vi "Set RfsaWlan Handle.vi"(8 "error in (no error)":errorcluster, 10 "RiviInstDriver Handle in":T1, 11 "niDTS WLAN INSTR TX in":refnum<class "niDTS WLAN INSTR TX.lvclass">) -> (0 "error out":errorcluster, 3 "niDTS WLAN INSTR TX out":refnum<class "niDTS WLAN INSTR TX.lvclass">)   [LabVIEW 2015, in "niDTS WLAN.lvlib" / "niDTS WLAN INSTR TX.lvclass"]
uses:
  niDTS WLAN INSTR TX.lvclass
  RiviInstDriver/niRfsaWlan/Includes/niRfsaWlan INC Handle.ctl
  RiviInstDriver/niRfsaWlan/Objects/niRfsaWlan.lvclass
  niDTS WLAN INSTR TX.lvclass/niDTS WLAN INSTR TX.ctl
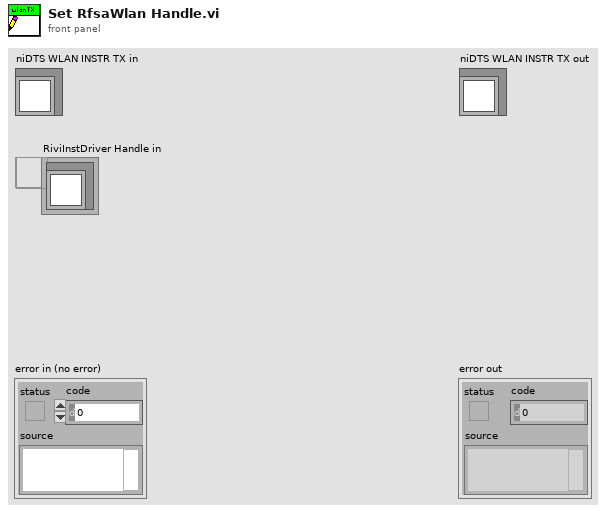
[diagram p1: front panel]
types:
  T1 = typedef "niRfsaWlan.lvclass/niRfsaWlan INC Handle.ctl" = refnum<data-value>
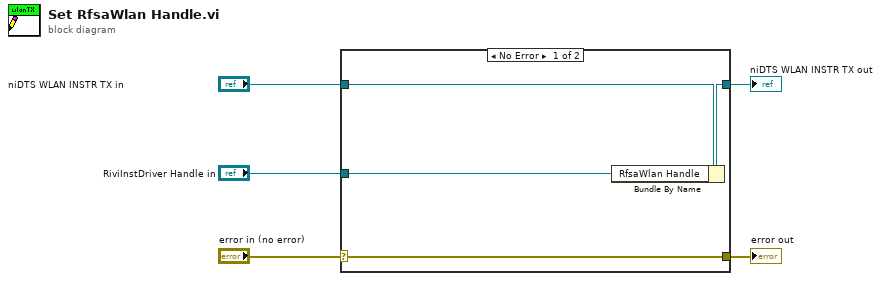
[diagram p0: block diagram]
diagram:
  n1 = case shown="No Error" "error in (no error)" {
    selector: "error in (no error)" -> [w9 w10]
    tunnel: [w9 w10] -> w4
    tunnel: [w7 w11] -> w2
    tunnel: "niDTS WLAN INSTR TX in" -> [w8 w11]
    tunnel: "RiviInstDriver Handle in" -> [w6 _]
    frame No Error {
      n2 = Bundle By Name(cluster=w8, "RfsaWlan Handle"=w6) -> (w7:refnum<class "niDTS WLAN INSTR TX.lvclass">)
    }
    frame Error {
    }
  }
  "error out" <- w4
  "niDTS WLAN INSTR TX out" <- w2
